vi "Set Active DUT Band Restrictions.vi"(6 "RX (None)":i32(ring) items=["None", "One", "Two"], 7 "TX (None)":i32(ring) items=["None", "One"], 8 "error in (no error)":errorcluster, 9 "Band Number (1)":i32=1, 10 "Band Type (LTE)":i32(ring) items=["LTE", "New Radio"], 11 "VISA resource name":refnum<visa-resource-name>) -> (0 "error out":errorcluster, 3 "VISA resource name out":refnum<visa-resource-name>)   [LabVIEW 2015, in "Rohde&Schwarz CMXP Base.lvlib"]
doc: "Configures restrictions for a frequency band assigned to connectors of the active DUT.\n\nAttribute:\n-\n\nRemote-control command:\n[CONFigure:]DUT:BAND:RESTrictions"
uses:
  <instrlib>/Rohde&Schwarz CMXP Base/Rohde&Schwarz CMXP Base.lvlib
  <instrlib>/Rohde&Schwarz CMXP Base/Private/rsidr_core.llb/rsidr_core.lvlib
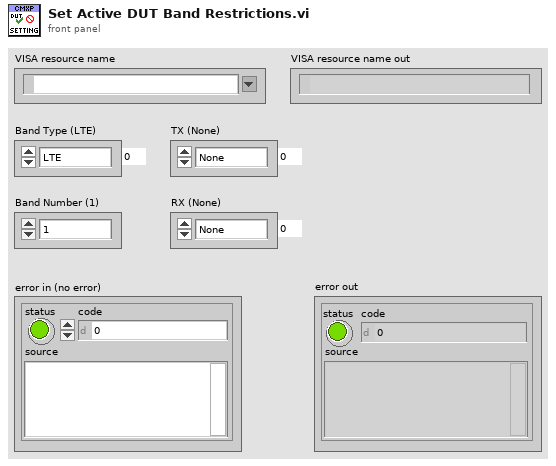
[diagram p1: front panel]
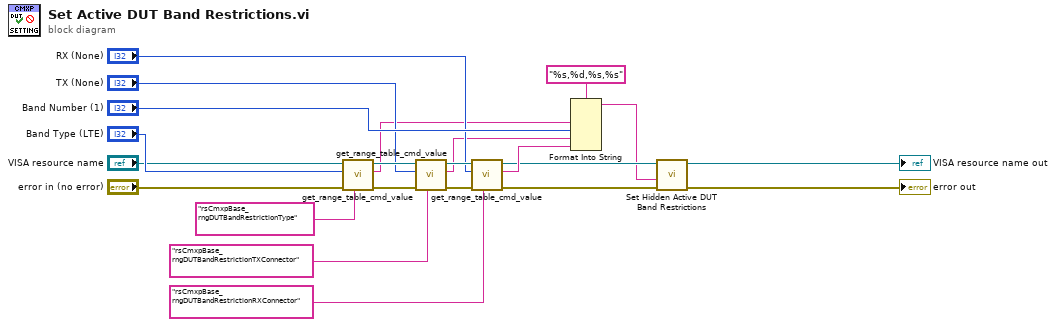
[diagram p0: block diagram]
diagram:
  n1 = call <instrlib>:"get_range_table_cmd_value.vi"("Range Table ID in"="rsCmxpBase_rngDUTBandRestrictionType", "error in"="error in (no error)", "Input Int32 value"="Band Type (LTE)", "VISA resource name"="VISA resource name") -> ("error out"=w18:errorcluster, "Cmd value out"=w5:string, "VISA resource name out"=w15:refnum<visa-resource-name>)  [unwired: 5 in]
  n2 = call <instrlib>:"get_range_table_cmd_value.vi"("Range Table ID in"="rsCmxpBase_rngDUTBandRestrictionTXConnector", "error in"=w18, "Input Int32 value"="TX (None)", "VISA resource name"=w15) -> ("error out"=w17:errorcluster, "Cmd value out"=w4:string, "VISA resource name out"=w16:refnum<visa-resource-name>)  [unwired: 5 in]
  n3 = call <instrlib>:"get_range_table_cmd_value.vi"("Range Table ID in"="rsCmxpBase_rngDUTBandRestrictionRXConnector", "error in"=w17, "Input Int32 value"="RX (None)", "VISA resource name"=w16) -> ("error out"=w6:errorcluster, "Cmd value out"=w3:string, "VISA resource name out"=w2:refnum<visa-resource-name>)  [unwired: 5 in]
  n4 = Format Into String(format string="%s,%d,%s,%s", w5, "Band Number (1)", w4, w3) -> (resulting string=w1:string)  [unwired: 2 in, 1 out]
  n5 = call "Set Hidden Active DUT Band Restrictions"("error in (no error)"=w6, "Hidden Active DUT Band Restrictions ()"=w1, "instrument handle"=w2) -> ("error out"=→"error out":errorcluster, "instrument handle out"=→"VISA resource name out":refnum<visa-resource-name>)  [unwired: 7 in]
